vi "Keithley 2260B Output DC Voltage and Current.vi"() -> ()   [LabVIEW 2009]
doc: "This example shows how to configure the instrument's output voltage level, over current protection, and over voltage protection. The actual voltage level and actual current level are returned as well as whether over voltage protection (OVP) or over current protection (OCP) has been tripped."
uses:
  <instrlib>/Keithley 2260B/Keithley 2260B.lvlib
panel:
  out "CC":bool
  out "CV":bool
  in  "OCP (5A)":dbl=5.0 format="%.3g"
  in  "Serial Configuration":T1={"Baud Rate"=9600, "Parity"=0, "Data Bits"=8, "Stop Bits"=10, "Flow Control"=0} {"Flow Control" items=["None", "XON/XOFF", "RTS/CTS", "XON/XOFF & RTS/CTS", "DTR/DSR", "XON/XOFF & DTR/DSR"]; "Stop Bits" items=["1.0"=10, "1.5"=15, "2.0"=20]; "Data Bits" items=["7"=7, "8"=8]; "Parity" items=["None", "Odd", "Even", "Mark", "Space"]; "Baud Rate" items=["300"=300, "600"=600, "1200"=1200, "2400"=2400, "4800"=4800, "9600"=9600, "19200"=19200]}
  in  "Stop Output":bool
  out "OCP Tripped?":bool
  out "OVP Tripped?":bool
  in  "OVP (10V)":dbl=10.0 format="%.3f"
  out "Actual Current Limit (A)":dbl format="%.3f"
  out "Actual Voltage Level (V)":dbl format="%.3f"
  in  "Voltage Level (0V)":dbl format="%.3f"
  in  "Current Level (0A)":dbl format="%.3f"
  in  "VISA resource name":refnum<visa-resource-name>
  # "Voltage"
  # "Current"
  # "WARNINGS: \nThe OVP, OCP Setting range depends on the 2260A Models\nFor 80V, the minimal value is 8V(10%). The max value is 88V(110%)\nFor 30V, the minimal value is 3V(10%). The max value is 33V(110%)\nFor 36A, the minimal value is 3.60A(10%). The max value is 39.6A(110%)"
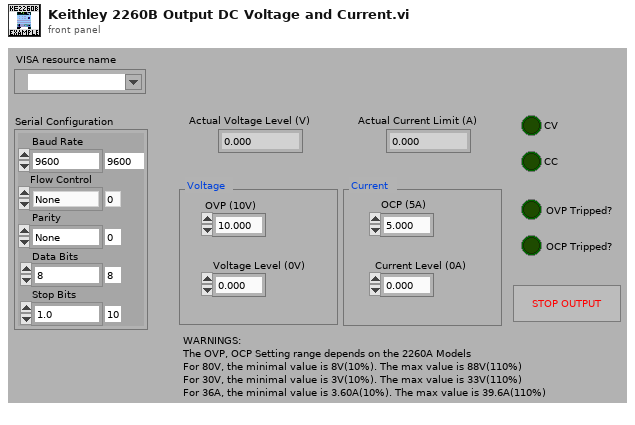
[diagram p1: front panel]
types:
  T1 = cluster{"Baud Rate":u32, "Parity":u16, "Data Bits":u16, "Stop Bits":u16, "Flow Control":u16}
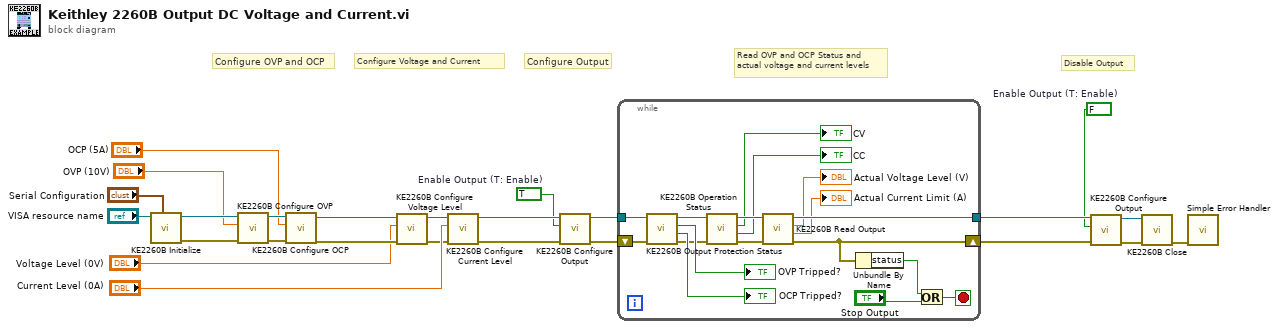
[diagram p0: block diagram]
diagram:
  w1 = FALSE  # Enable Output (T: Enable)
  w2 = TRUE  # Enable Output (T: Enable)
  # "Configure Voltage and Current"
  # "Disable Output"
  # "Read OVP and OCP Status and\nactual voltage and current levels"
  # "Configure Output"
  # "Configure OVP and OCP"
  n1 = call <instrlib>:"KE2260B Initialize.vi"("Serial Configuration"="Serial Configuration", "VISA resource name"="VISA resource name") -> ("error out"=w16:errorcluster, "VISA resource name out"=w17:refnum<visa-resource-name>)  [unwired: 8 in]
  n2 = call <instrlib>:"KE2260B Configure OVP.vi"("error in (no error)"=w16, "OVP (0.000 V)"="OVP (10V)", "VISA resource name"=w17) -> ("error out"=w13:errorcluster, "VISA resource name out"=w12:refnum<visa-resource-name>)  [unwired: 7 in]
  n3 = call <instrlib>:"KE2260B Configure OCP.vi"("error in (no error)"=w13, "OCP (0.000 V)"="OCP (5A)", "VISA resource name"=w12) -> ("error out"=w9:errorcluster, "VISA resource name out"=w10:refnum<visa-resource-name>)  [unwired: 7 in]
  n4 = call <instrlib>:"KE2260B Configure Voltage Level.vi"("error in (no error)"=w9, "Voltage Level (0.000 V)"="Voltage Level (0V)", "VISA resource name"=w10) -> ("error out"=w5:errorcluster, "VISA resource name out"=w6:refnum<visa-resource-name>)  [unwired: 7 in]
  n5 = call <instrlib>:"KE2260B Configure Current Level.vi"("error in (no error)"=w5, "Current Level (0.000 A)"="Current Level (0A)", "VISA resource name"=w6) -> ("error out"=w3:errorcluster, "VISA resource name out"=w4:refnum<visa-resource-name>)  [unwired: 7 in]
  n6 = call <instrlib>:"KE2260B Configure Output.vi"("error in (no error)"=w3, "Enable Output (T: Enable)"=w2, "VISA resource name"=w4) -> ("error out"=w23:errorcluster, "VISA resource name out"=w24:refnum<visa-resource-name>)  [unwired: 7 in]
  n7 = while {
    tunnel: w24 -> [w42]
    tunnel: [w40] -> w22
    shift-right: [w33] -> w21
    shift-left: w23 -> [w41]
    stop <- w35 stop-if-true
    n8 = call <instrlib>:"KE2260B Output Protection Status.vi"("error in (no error)"=w41, "VISA resource name"=w42) -> ("error out"=w30:errorcluster, "OCP Tripped?"=→"OCP Tripped?":bool, "OVP Tripped?"=→"OVP Tripped?":bool, "VISA resource name out"=w31:refnum<visa-resource-name>)  [unwired: 6 in]
    n9 = call <instrlib>:"KE2260B Operation Status.vi"("error in (no error)"=w30, "VISA resource name"=w31) -> ("error out"=w28:errorcluster, "CC"=→"CC":bool, "CV"=→"CV":bool, "VISA resource name out"=w29:refnum<visa-resource-name>)  [unwired: 4 in, 2 out]
    n10 = call <instrlib>:"KE2260B Read Output.vi"("error in (no error)"=w28, "VISA resource name"=w29) -> ("error out"=w33:errorcluster, "Actual Current Level (A)"=→"Actual Current Limit (A)":dbl, "Actual Voltage Level (V)"=→"Actual Voltage Level (V)":dbl, "VISA resource name out"=w40:refnum<visa-resource-name>)  [unwired: 6 in]
    n11 = Unbundle By Name(w33) -> ("status"=w32:bool)
    n12 = Or(x=w32, y="Stop Output") -> (x .or. y?=w35:bool)
  }
  n13 = call <instrlib>:"KE2260B Configure Output.vi"("error in (no error)"=w21, "Enable Output (T: Enable)"=w1, "VISA resource name"=w22) -> ("error out"=w19:errorcluster, "VISA resource name out"=w20:refnum<visa-resource-name>)  [unwired: 7 in]
  n14 = call <instrlib>:"KE2260B Close.vi"("error in (no error)"=w19, "VISA resource name"=w20) -> ("error out"=w18:errorcluster)  [unwired: 9 in]
  n15 = call <vilib>:"Simple Error Handler.vi"("error in (no error)"=w18) -> ()  [unwired: 4 in, 5 out]
